vi "通讯配置.vi"(8 "error in (no error)":errorcluster caption="错误输入（无错误）", 11 "MainPage 输入":refnum<class "MainPage.lvclass">) -> (0 "error out":errorcluster caption="错误输出")   [LabVIEW 2019, in "MainPage.lvlib" / "MainPage.lvclass"]
uses:
  MainPage.lvclass
  MainPage.lvclass/MainPage.ctl
panel:
  out "客服端参数":cluster{"本机端口":u16, "主机 IP":string, "主机端口":u16}={"本机端口"=0, "主机 IP"="0", "主机端口"=0}
  out "服务端参数":cluster{"本机 IP":string, "侦听端口":u16}
  out "串口参数":T1={"VISA串口名称"="", "波特率"=9600, "停止位"=10, "流控制"=0, "数据位"=8, "奇偶校验"=enum."None", "超时"=2000, "启用终止符？"=FALSE, "终止符"=10} {"终止符" format="%.0x"; "数据位" min=5 max=8 step=1; "流控制" items=["无", "XON/XOFF", "RTS/CTS", "XON/XOFF & RTS/CTS", "DTR/DSR", "XON/XOFF & DTR/DSR"]; "停止位" items=["1.0"=10, "1.5"=15, "2.0"=20]; "波特率" items=["9600"=9600, "115200"=15]}
  in  "服务侦听":bool
  # "模式切换 全部清除\n模式不变-判断内容是否改变"
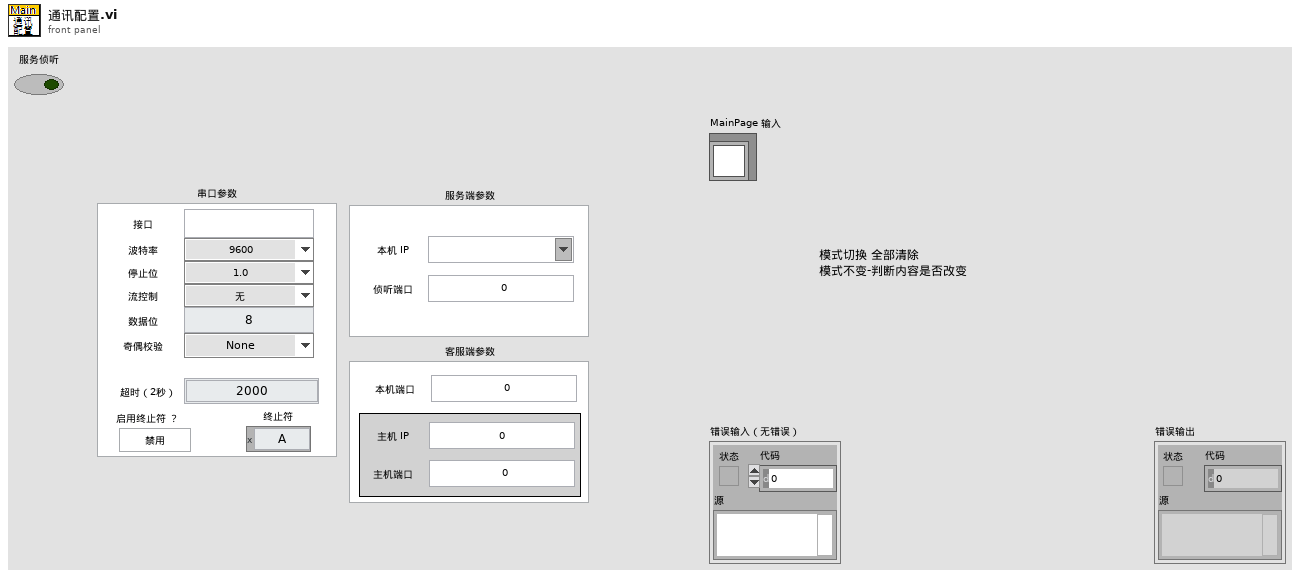
[diagram p1: front panel]
types:
  T1 = cluster{"VISA串口名称":refnum<visa-resource-name>, "波特率":u32, "停止位":u16, "流控制":u16, "数据位":u16, "奇偶校验":enum16{"None", "Odd", "Even", "Mark", "Space"}, "超时":u32, "启用终止符？":bool, "终止符":u8}
  T2 = cluster{"客服端识别.客P-主IP:Port":string, "连接ID":refnum<k5>}
  T3 = cluster{"连接ID":refnum<k5>, "服务端识别.本机IP":string, "服务端识别.本机端口":u16}
  T4 = enum16{"INI", "获取数据", "连接方式更新", "串口更新", "服务端当前目标", "服务端识别及ID", "客服端识别", "ID记录增加", "ID记录删除", "ID记录重置"}
  T5 = typedef "MainPage.lvlib/MainPage.lvclass/DataRef_通讯接口-弃用.ctl" = cluster{"连接方式":enum16{"串口", "网口(客服端)", "网口(服务端)"}, "VISA串口名称":refnum<visa-resource-name>, "服务端识别":cluster{"本机IP":string, "本机端口":u16, "当前目标":string, "服务端侦听ID":refnum<k5>}, "客服端识别":cluster{"客P-主IP:Port":string}, "ID记录":map{string, refnum<k5>}}
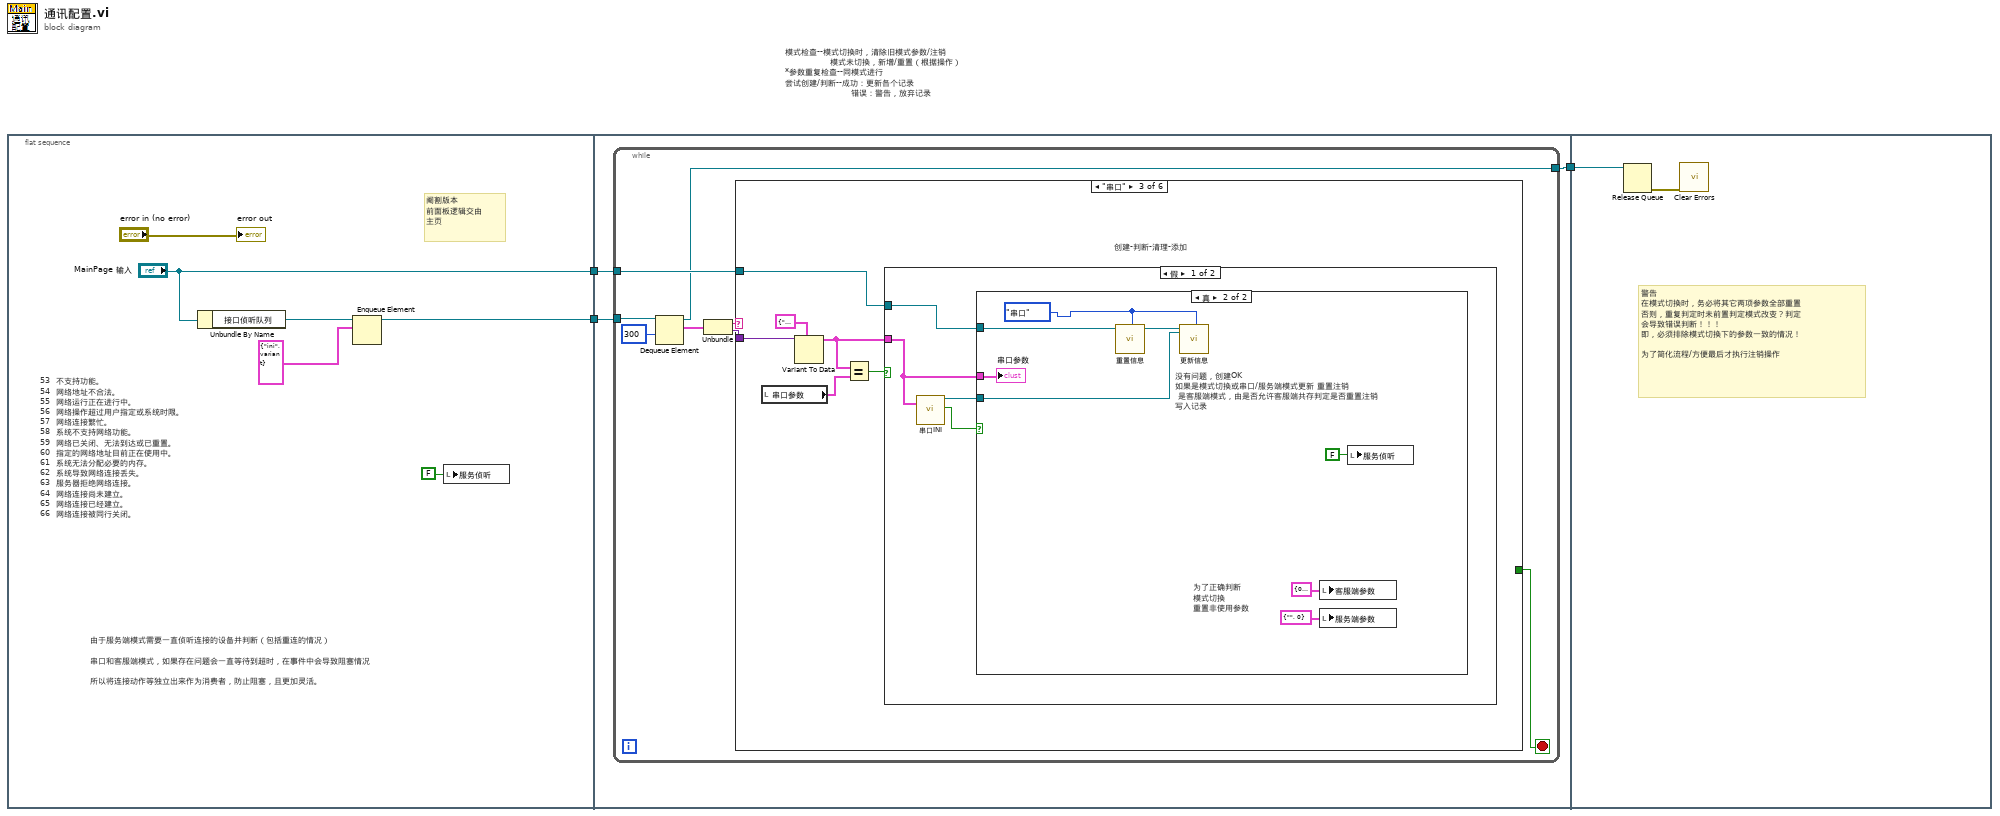
[diagram p0: block diagram]
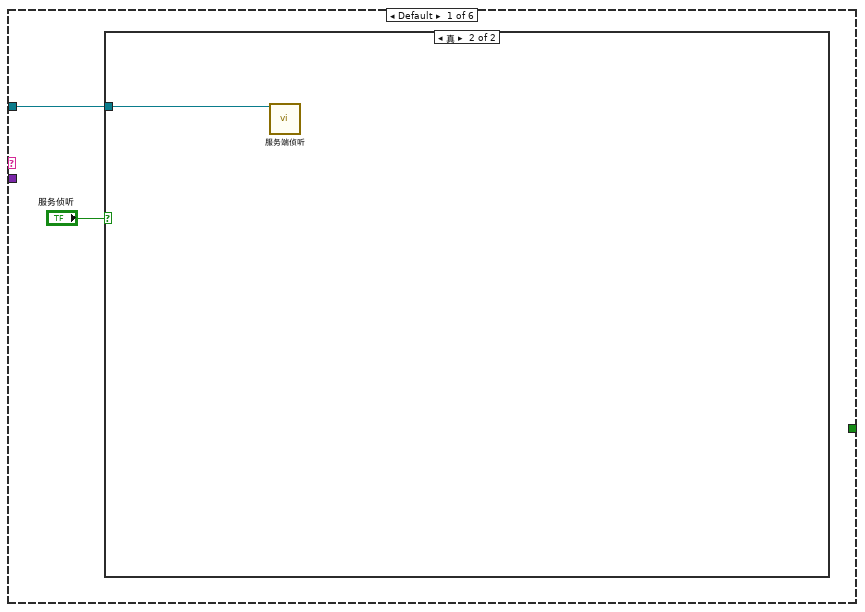
[diagram p2: hidden frame]
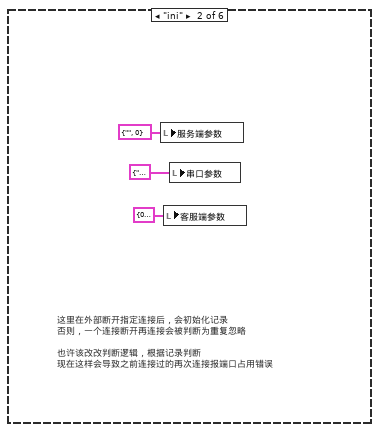
[diagram p4: hidden frame]
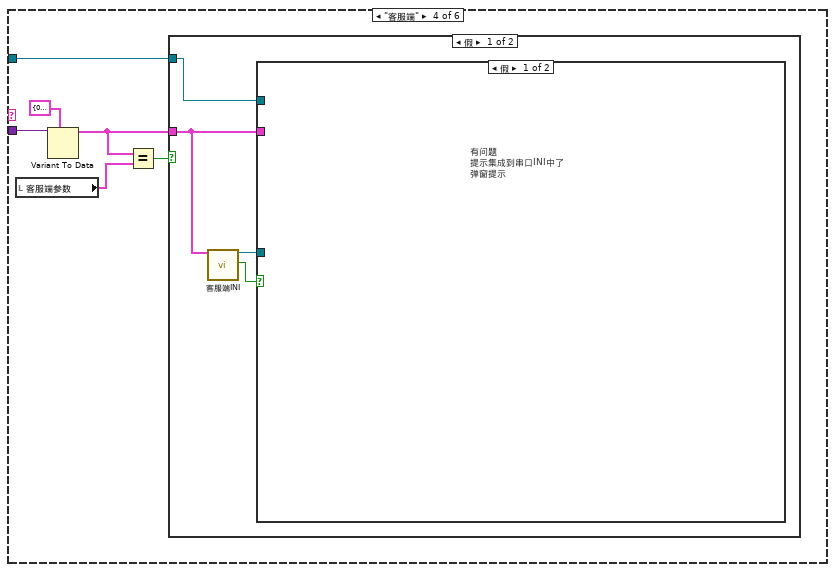
[diagram p7: hidden frame]
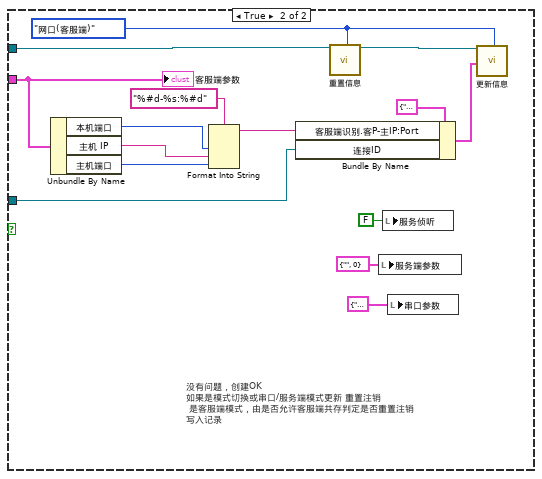
[diagram p8: hidden frame]
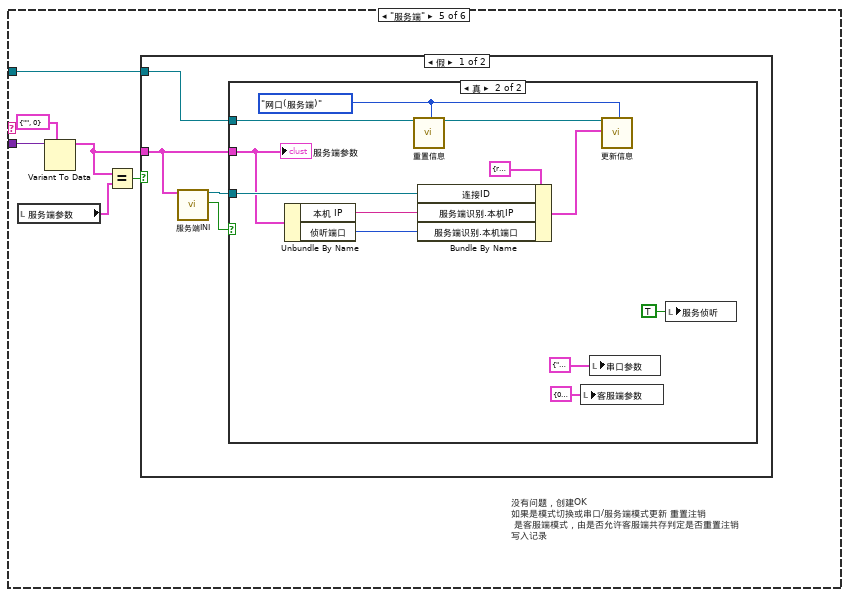
[diagram p10: hidden frame]
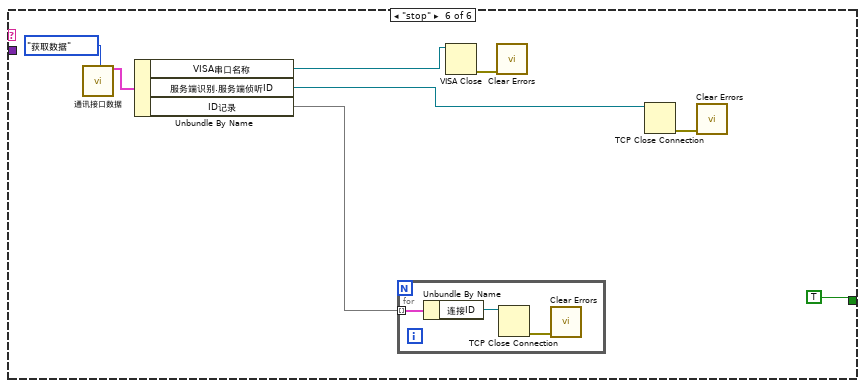
[diagram p13: hidden frame]
diagram:
  # "模式检查--模式切换时，清除旧模式参数/注销\n               模式未切换，新增/重置（根据操作）\n*参数重复检查--同模式进行\n尝试创建/判断--成功：更新各个记录\n                      错误：警告，放弃记录"
  n1 = flat-sequence {
    tunnel: [w9] -> w3
    tunnel: ["MainPage 输入"] -> w1
    tunnel: w3 -> [w10]
    tunnel: [w12] -> w2
    tunnel: w1 -> [w11]
    tunnel: w2 -> [w104]
    frame #0 {
      # "53  不支持功能。\n54  网络地址不合法。\n55  网络运行正在进行中。\n56  网络操作超过用户指定或系统时限。\n57  网络连接繁忙。\n58  系统不支持网络功能。\n59  网络已关闭、无法到达或已重置。\n60  指定的网络地址目前正在使用中。\n61  系统无法分配必要的内存。\n62  系统导致网络连接丢失。\n63  服务器拒绝网络连接。\n64  网络连接尚未建立。\n65  网络连接已经建立。\n66  网络连接被同行关闭。"
      # "阉割版本\n前面板逻辑交由\n主页"
      # "由于服务端模式需要一直侦听连接的设备并判断（包括重连的情况）\n\n串口和客服端模式，如果存在问题会一直等待到超时，在事件中会导致阻塞情况\n\n所以将连接动作等独立出来作为消费者，防止阻塞，且更加灵活。"
      n2 = Unbundle By Name("MainPage 输入") -> ("接口侦听队列"=w6:refnum<queue>)
      n3 = Enqueue Element(queue=w6, element=cluster{string, variant} {"ini", variant} ("元素")) -> (queue out=w9:refnum<queue>)  [unwired: 2 in, 2 out]
      n4 = local write "服务侦听"(FALSE ("服务侦听")) -> ()
      "error out" <- "error in (no error)"
    }
    frame #1 {
      n5 = while {
        tunnel: w10 -> [w20]
        tunnel: [w13] -> w12
        tunnel: w11 -> [w14]
        stop <- w16 stop-if-true
        n6 = Dequeue Element(queue=w20, timeout in ms (-1)=300 ("超时毫秒(-1)")) -> (queue out=w13:refnum<queue>, element=w15:cluster{string, variant})  [unwired: 1 in, 2 out]
        n7 = Unbundle(w15) -> (w18:string, w17:variant)
        n8 = case shown="\"串口\"" w18 {
          tunnel: w17 -> [_ _ w32 w50 w75 _]
          tunnel: [_ _ _ _ _ TRUE] -> w16
          tunnel: w14 -> [w21 _ w27 w48 w73 _]
          frame Default {
            n9 = case shown="真" "服务侦听" {
              tunnel: w21 -> [_ w23]
              frame False {
                # "非服务端模式，不需要一直侦听"
              }
              frame True {
                n10 = call "服务端侦听.vi"("MainPage 输入"=w23) -> ()  [unwired: 18 in, 1 out]
              }
            }
          }
          frame "ini" {
            # "这里在外部断开指定连接后，会初始化记录\n否则，一个连接断开再连接会被判断为重复忽略\n\n也许该改改判断逻辑，根据记录判断\n现在这样会导致之前连接过的再次连接报端口占用错误"
            n11 = local write "服务端参数"(cluster{"本机 IP":string, "侦听端口":u16} {"本机 IP"="", "侦听端口"=0} ("服务端参数")) -> ()
            n12 = local write "客服端参数"(cluster{"本机端口":u16, "主机 IP":string, "主机端口":u16} {"本机端口"=0, "主机 IP"="0", "主机端口"=0} ("客服端参数")) -> ()
            n13 = local write "串口参数"(T1 {"VISA串口名称"="", "波特率"=9600, "停止位"=10, "流控制"=0, "数据位"=0, "奇偶校验"=enum."None", "超时"=0, "启用终止符？"=FALSE, "终止符"=0} ("串口参数")) -> ()
          }
          frame "串口" {
            # "创建-判断-清理-添加"
            n14 = local read "串口参数"() -> (w30:T1)
            n15 = Variant To Data(type=T1 {"VISA串口名称"="", "波特率"=9600, "停止位"=10, "流控制"=0, "数据位"=8, "奇偶校验"=enum."None", "超时"=2000, "启用终止符？"=FALSE, "终止符"=10} ("串口参数"), Variant=w32) -> (data=w28:T1)  [unwired: 1 in, 1 out]
            n16 = Equal?(x=w28, y=w30) -> (x = y?=w29:bool)
            n17 = case shown="假" w29 {
              tunnel: w28 -> [w33 _]
              tunnel: w27 -> [w34 _]
              frame False {
                n18 = call "串口INI.vi"("串口参数"=w33) -> ("串口"=w35:refnum<visa-resource-name>, "可用？"=w36:bool)  [unwired: 17 in]
                n19 = case shown="真" w36 {
                  tunnel: w35 -> [_ w41]
                  tunnel: w34 -> [_ w44]
                  tunnel: w33 -> [_ w43]
                  frame False {
                    # "有问题\n提示集成到串口INI中了\n弹窗提示"
                  }
                  frame True {
                    w37 = enum16{"串口", "网口(客服端)", "网口(服务端)"}."串口" ("连接方式")
                    # "为了正确判断\n模式切换\n重置非使用参数"
                    # "没有问题，创建OK\n如果是模式切换或串口/服务端模式更新 重置注销\n 是客服端模式，由是否允许客服端共存判定是否重置注销\n写入记录"
                    n20 = call "重置信息.vi"("MainPage 输入"=w44, "连接方式"=w37) -> ("MainPage 输出"=w42:refnum<class "MainPage.lvclass">)  [unwired: 17 in]
                    n21 = call "更新信息.vi"("MainPage 输入"=w42, "VISA串口名称"=w41, "连接方式"=w37) -> ()  [unwired: 15 in, 2 out]
                    n22 = local write "客服端参数"(cluster{"本机端口":u16, "主机 IP":string, "主机端口":u16} {"本机端口"=0, "主机 IP"="0", "主机端口"=0} ("客服端参数")) -> ()
                    n23 = local write "服务端参数"(cluster{"本机 IP":string, "侦听端口":u16} {"本机 IP"="", "侦听端口"=0} ("服务端参数")) -> ()
                    n24 = local write "服务侦听"(FALSE ("服务侦听")) -> ()
                    "串口参数" <- w43
                  }
                }
              }
              frame True {
                # "默认排除了模式切换时值相同的情况(模式切换时数据记录全部重置)\n\n这里处理的就只有重复确认的操作了"
              }
            }
          }
          frame "客服端" {
            n25 = local read "客服端参数"() -> (w47:cluster{"本机端口":u16, "主机 IP":string, "主机端口":u16})
            n26 = Variant To Data(type=cluster{"本机端口":u16, "主机 IP":string, "主机端口":u16} {"本机端口"=0, "主机 IP"="", "主机端口"=0} ("客服端参数"), Variant=w50) -> (data=w45:cluster{"本机端口":u16, "主机 IP":string, "主机端口":u16})  [unwired: 1 in, 1 out]
            n27 = Equal?(x=w45, y=w47) -> (x = y?=w46:bool)
            n28 = case shown="假" w46 {
              tunnel: w48 -> [w54 _]
              tunnel: w45 -> [w53 _]
              frame False {
                n29 = call "客服端INI.vi"("客服端参数"=w53) -> ("连接ID"=w51:refnum<k5>, "可用？"=w52:bool)  [unwired: 17 in]
                n30 = case shown="假" w52 {
                  tunnel: w54 -> [_ w69]
                  tunnel: w53 -> [_ w62]
                  tunnel: w51 -> [_ w61]
                  frame False {
                    # "有问题\n提示集成到串口INI中了\n弹窗提示"
                  }
                  frame True {
                    w55 = enum16{"串口", "网口(客服端)", "网口(服务端)"}."网口(客服端)" ("连接方式")
                    # "没有问题，创建OK\n如果是模式切换或串口/服务端模式更新 重置注销\n 是客服端模式，由是否允许客服端共存判定是否重置注销\n写入记录"
                    n31 = Unbundle By Name(w62) -> ("本机端口"=w59:u16, "主机 IP"=w58:string, "主机端口"=w57:u16)
                    n32 = Format Into String(format string="%#d-%s:%#d" ("格式字符串"), w59, w58, w57) -> (resulting string=w56:string)  [unwired: 2 in, 1 out]
                    n33 = Bundle By Name(cluster=T2 {"客服端识别.客P-主IP:Port"="", "连接ID"=refnum} ("客服端"), "客服端识别.客P-主IP:Port"=w56, "连接ID"=w61) -> (w63:T2)
                    n34 = call "重置信息.vi"("MainPage 输入"=w69, "连接方式"=w55) -> ("MainPage 输出"=w68:refnum<class "MainPage.lvclass">)  [unwired: 17 in]
                    n35 = local write "服务端参数"(cluster{"本机 IP":string, "侦听端口":u16} {"本机 IP"="", "侦听端口"=0} ("服务端参数")) -> ()
                    n36 = local write "服务侦听"(FALSE ("服务侦听")) -> ()
                    n37 = local write "串口参数"(T1 {"VISA串口名称"="", "波特率"=9600, "停止位"=10, "流控制"=0, "数据位"=0, "奇偶校验"=enum."None", "超时"=0, "启用终止符？"=FALSE, "终止符"=0} ("串口参数")) -> ()
                    n38 = call "更新信息.vi"("MainPage 输入"=w68, "客服端"=w63, "连接方式"=w55) -> ()  [unwired: 15 in, 2 out]
                    "客服端参数" <- w62
                  }
                }
              }
              frame True {
              }
            }
          }
          frame "服务端" {
            # "没有问题，创建OK\n如果是模式切换或串口/服务端模式更新 重置注销\n 是客服端模式，由是否允许客服端共存判定是否重置注销\n写入记录"
            n39 = local read "服务端参数"() -> (w72:cluster{"本机 IP":string, "侦听端口":u16})
            n40 = Variant To Data(type=cluster{"本机 IP":string, "侦听端口":u16} {"本机 IP"="", "侦听端口"=0} ("服务端参数 2"), Variant=w75) -> (data=w71:cluster{"本机 IP":string, "侦听端口":u16})  [unwired: 1 in, 1 out]
            n41 = Equal?(x=w71, y=w72) -> (x = y?=w70:bool)
            n42 = case shown="假" w70 {
              tunnel: w73 -> [w79 _]
              tunnel: w71 -> [w78 _]
              frame False {
                n43 = call "服务端INI.vi"("服务端配置"=w78) -> ("侦听ID"=w76:refnum<k5>, "可用？"=w77:bool)  [unwired: 17 in]
                n44 = case shown="真" w77 {
                  tunnel: w79 -> [_ w91]
                  tunnel: w78 -> [_ w86]
                  tunnel: w76 -> [_ w88]
                  frame False {
                    # "有问题\n提示集成到串口INI中了\n弹窗提示"
                  }
                  frame True {
                    w80 = enum16{"串口", "网口(客服端)", "网口(服务端)"}."网口(服务端)" ("连接方式")
                    n45 = Unbundle By Name(w86) -> ("本机 IP"=w85:string, "侦听端口"=w84:u16)
                    n46 = call "重置信息.vi"("MainPage 输入"=w91, "连接方式"=w80) -> ("MainPage 输出"=w90:refnum<class "MainPage.lvclass">)  [unwired: 17 in]
                    n47 = Bundle By Name(cluster=T3 {"连接ID"=refnum, "服务端识别.本机IP"="", "服务端识别.本机端口"=0} ("服务端"), "连接ID"=w88, "服务端识别.本机IP"=w85, "服务端识别.本机端口"=w84) -> (w87:T3)
                    n48 = local write "客服端参数"(cluster{"本机端口":u16, "主机 IP":string, "主机端口":u16} {"本机端口"=0, "主机 IP"="0", "主机端口"=0} ("客服端参数")) -> ()
                    n49 = local write "串口参数"(T1 {"VISA串口名称"="", "波特率"=9600, "停止位"=10, "流控制"=0, "数据位"=0, "奇偶校验"=enum."None", "超时"=0, "启用终止符？"=FALSE, "终止符"=0} ("串口参数")) -> ()
                    n50 = call "更新信息.vi"("MainPage 输入"=w90, "服务端"=w87, "连接方式"=w80) -> ()  [unwired: 15 in, 2 out]
                    n51 = local write "服务侦听"(TRUE ("服务侦听")) -> ()
                    "服务端参数" <- w86
                  }
                }
              }
              frame True {
              }
            }
          }
          frame "stop" {
            n52 = call "通讯接口数据.vi"("枚举"=T4."获取数据") -> ("通讯接口数据"=w93:T5)  [unwired: 18 in]
            n53 = Unbundle By Name(w93) -> ("VISA串口名称"=w97:refnum<visa-resource-name>, "服务端识别.服务端侦听ID"=w95:refnum<k5>, "ID记录"=w94:map{string, refnum<k5>})
            n54 = for {
              tunnel: w94 -> [w101] mode=indexing
              n55 = Unbundle By Name(w101) -> ("连接ID"=w100:refnum<k5>)
              n56 = TCP Close Connection(connection ID=w100) -> (error out=w102:errorcluster)  [unwired: 2 in, 1 out]
              n57 = call <vilib>:"Clear Errors.vi"("error in (no error)"=w102) -> ()  [unwired: 5 in, 2 out]
            }
            n58 = VISA Close(VISA resource name=w97) -> (error out=w98:errorcluster)  [unwired: 1 in]
            n59 = call <vilib>:"Clear Errors.vi"("error in (no error)"=w98) -> ()  [unwired: 5 in, 2 out]
            n60 = TCP Close Connection(connection ID=w95) -> (error out=w96:errorcluster)  [unwired: 2 in, 1 out]
            n61 = call <vilib>:"Clear Errors.vi"("error in (no error)"=w96) -> ()  [unwired: 5 in, 2 out]
          }
        }
      }
    }
    frame #2 {
      # "警告\n在模式切换时，务必将其它两项参数全部重置\n否则，重复判定时未前置判定模式改变？判定\n会导致错误判断！！！\n即，必须排除模式切换下的参数一致的情况！\n\n为了简化流程/方便最后才执行注销操作"
      n62 = Release Queue(queue=w104) -> (error out=w103:errorcluster)  [unwired: 2 in, 2 out]
      n63 = call <vilib>:"Clear Errors.vi"("error in (no error)"=w103) -> ()  [unwired: 5 in, 2 out]
    }
  }
